vi "Get configuration chain.vi"(8 "error in (no error)":errorcluster, 11 "GalvoBase in":refnum<class "ImagingModeSPIM.lvclass">) -> (0 "error out":errorcluster, 1 "class name":string[](array[string]), 2 "configuration chain":variant[](array[variant]), 3 "GalvoBase out":refnum<class "ImagingModeSPIM.lvclass">)   [LabVIEW 2012, in "ImagingModeSPIM.lvclass"]
doc: "Returns an array of variants containing the configuration clusters of each class in the inheritance chain (lowest child class first), together with an array of all class names in the inheritance chain.\n\nFor classes without configuration cluster, the configuration chain contains empty variants."
uses:
  ImagingModeSPIM.lvclass
  <vilib>/Distrio/Murmex/Murmex/Murmex.lvclass
  ImagingModeSPIM.lvclass/ImagingModeSPIM.ctl
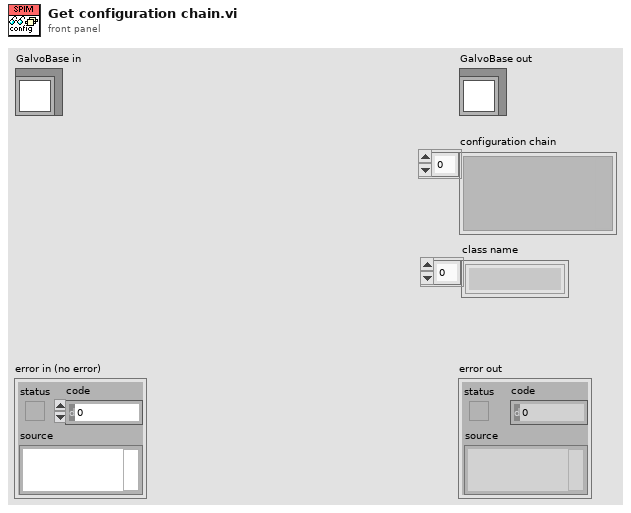
[diagram p1: front panel]
types:
  T1 = typedef "ImagingModeSPIM.lvclass/configuration_cluster.ctl" = cluster{"Sampling rate":dbl, "Samples per channel":i32, "Number of channels":T2, "Task cluster":T3}
  T2 = typedef "ImagingModeSPIM.lvclass/number of channels.ctl" = enum16{"empty", "double sided + PC", "double sided + WFS"}
  T3 = typedef "ImagingModeSPIM.lvclass/task_cluster.ctl" = cluster{"min Voltage":dbl[unit], "max Voltage":dbl[unit], "physical channel":string}
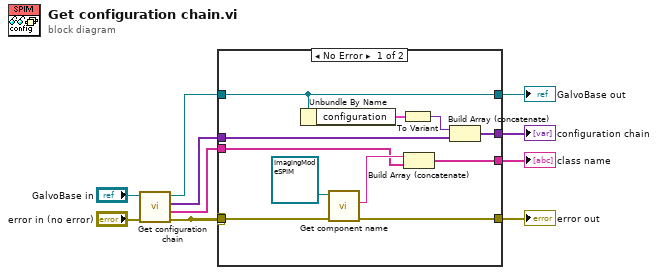
[diagram p0: block diagram]
diagram:
  n1 = call-parent "Get configuration chain.vi"("error in (no error)"="error in (no error)", "MurmexBase in"="GalvoBase in") -> ("error out"=w3:errorcluster, "class name"=w6:string[], "configuration chain"=w8:variant[], "MurmexBase out"=w2:refnum<class "ImagingModeSPIM.lvclass">)  [unwired: 6 in]
  n2 = case shown="No Error" w3 {
    selector: w3 -> [_ w23]
    tunnel: w8 -> [w19 w24]
    tunnel: [w18 w24] -> w7
    tunnel: w6 -> [w16 w22]
    tunnel: [w15 w22] -> w5
    tunnel: w2 -> [w11 w25]
    tunnel: w3 -> [w13 _]
    tunnel: [w12 w23] -> w4
    tunnel: [w11 w25] -> w1
    frame No Error {
      n3 = Unbundle By Name(w11) -> ("configuration"=w21:T1)
      n4 = call <vilib>:"Get component name.vi"("error in (no error)"=w13, "Murmex in"=refnum<class "ImagingModeSPIM.lvclass"> refnum ("Galvo.lvclass")) -> ("error out"=w12:errorcluster, "component name"=w17:string)  [unwired: 7 in, 1 out]
      n5 = To Variant(anything=w21) -> (Variant=w20:variant)
      n6 = Build Array (concatenate)(w17, w16) -> (w15:string[])
      n7 = Build Array (concatenate)(w20, w19) -> (w18:variant[])
    }
    frame Error {
    }
  }
  "error out" <- w4
  "GalvoBase out" <- w1
  "configuration chain" <- w7
  "class name" <- w5
